vi "dynamicStartProcessVI.vi"(8 "error in (no error)":errorcluster) -> (0 "error out":errorcluster, 3 "VI out":refnum<vi>)   [LabVIEW 2013, in "main.lvlib"]
uses:
  main.lvlib
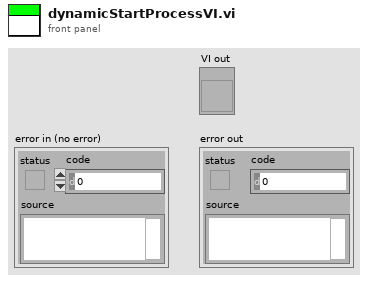
[diagram p1: front panel]
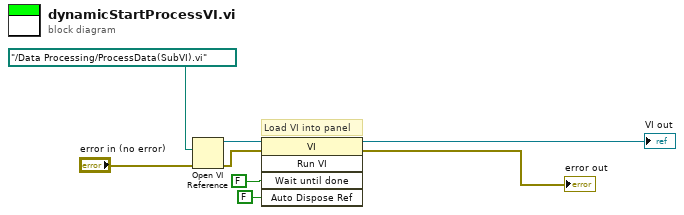
[diagram p0: block diagram]
diagram:
  # "Load VI into panel"
  n1 = Open VI Reference(vi path=path "../Data Processing/ProcessData(SubVI).vi", error in (no error)="error in (no error)") -> (vi reference=w1:refnum<vi>, error out=w7:errorcluster)  [unwired: 4 in]
  n2 = invoke class="VI" method="Run VI"(reference=w1, error in=w7, "Wait until done"=FALSE ("Wait Until Done"), "Auto Dispose Ref"=FALSE ("Auto Dispose Reference")) -> (reference out=→"VI out":refnum<vi>, error out=→"error out":errorcluster)  [unwired: 1 in, 3 out]
